vi "test-ramsete.vi"() -> (3 "AtReference End":bool)   [LabVIEW 2019]
uses:
  <vilib>/Rock Robotics/WPI/ThirdParty/JAS_Junk/TrajLib/CHASSIS_SPEEDS.ctl
  <vilib>/Rock Robotics/WPI/ThirdParty/JAS_Junk/TrajLib/POSE2D.ctl
  <vilib>/Rock Robotics/WPI/ThirdParty/JAS_Junk/TrajLib/TRANSLATION2D.ctl
  <vilib>/Rock Robotics/WPI/ThirdParty/JAS_Junk/TrajLib/ROTATION2D.ctl
  <vilib>/Rock Robotics/WPI/ThirdParty/JAS_Junk/TrajLib/TRAJ_STATE.ctl
  <vilib>/Rock Robotics/WPI/ThirdParty/JAS_Junk/TrajLib/TRAJECTORY.ctl
  <vilib>/Rock Robotics/WPI/ThirdParty/JAS_Junk/TrajLib/Rotation_CreateAngle.vi
  <vilib>/Rock Robotics/WPI/ThirdParty/JAS_Junk/TrajLib/Translation_Create.vi
  <vilib>/Rock Robotics/WPI/ThirdParty/JAS_Junk/TrajLib/Trajectory_Library.lvlib
panel:
  out "AtReference":bool
  out "out POSe":T1 {"ROTATION"."SIN" format="%13.4f"; "ROTATION"."COS" format="%13.4f"; "ROTATION"."VALUE" format="%13.4f"; "TRANSLATION"."Y" format="%14.3f"; "TRANSLATION"."X" format="%14.3f"}
  out "TRAJECTORY":T4 {"States"."POSE"."ROTATION"."SIN" format="%13.4f"; "States"."POSE"."ROTATION"."COS" format="%13.4f"; "States"."POSE"."ROTATION"."VALUE" format="%13.4f"; "States"."POSE"."TRANSLATION"."Y" format="%14.3f"; "States"."POSE"."TRANSLATION"."X" format="%14.3f"; "TotalTImeSecs" format="%20.3f"}
  out "OutputTRAJ_STATE":T5={"TimeSeconds"=0.0, "Velocity"=0.0, "Acceleration"=0.0, "POSE"={"TRANSLATION"={"X"=0.0, "Y"=0.0}, "ROTATION"={"VALUE"=0.0, "COS"=1.0, "SIN"=0.0}}, "Curvature"=0.0} {"POSE"."ROTATION"."SIN" format="%13.4f"; "POSE"."ROTATION"."COS" format="%13.4f"; "POSE"."ROTATION"."VALUE" format="%13.4f"; "POSE"."TRANSLATION"."Y" format="%14.3f"; "POSE"."TRANSLATION"."X" format="%14.3f"}
  out "Integer":i32
  out "UpdatedPose":T1 {"ROTATION"."SIN" format="%13.4f"; "ROTATION"."COS" format="%13.4f"; "ROTATION"."VALUE" format="%13.4f"; "TRANSLATION"."Y" format="%14.3f"; "TRANSLATION"."X" format="%14.3f"}
  out "CHASSIS Speeds":T6 {"vOmega" format="%10.3f"; "vY" format="%10.3f"; "vX" format="%10.3f"}
  out "Samp-int":i32
  out "Samp-real":dbl
  # "Ramsete"
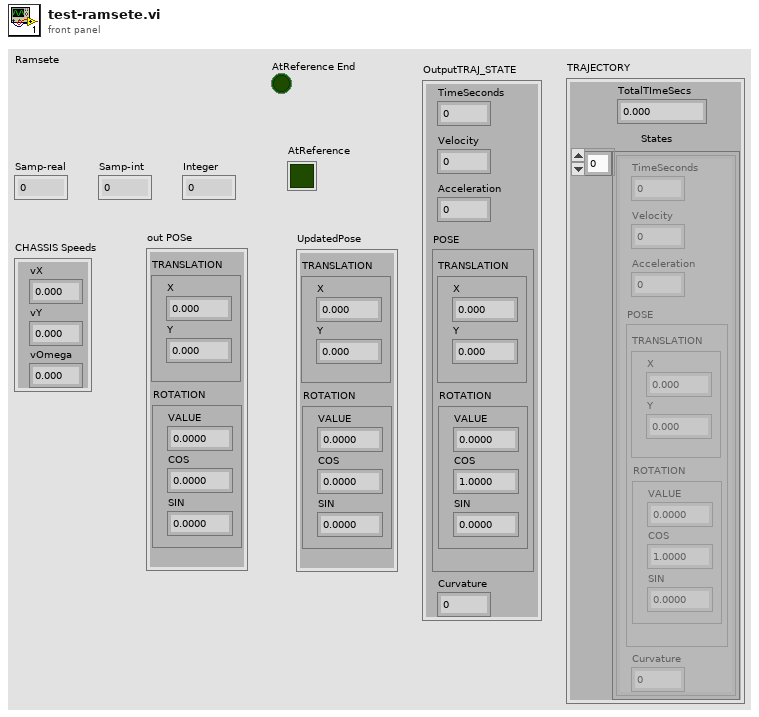
[diagram p1: front panel]
types:
  T1 = typedef "Trajectory_Library.lvlib/POSE2D.ctl" = cluster{"TRANSLATION":T2, "ROTATION":T3}
  T2 = typedef "Trajectory_Library.lvlib/TRANSLATION2D.ctl" = cluster{"X":dbl, "Y":dbl}
  T3 = typedef "Trajectory_Library.lvlib/ROTATION2D.ctl" = cluster{"VALUE":dbl, "COS":dbl, "SIN":dbl}
  T4 = typedef "Trajectory_Library.lvlib/TRAJECTORY.ctl" = cluster{"TotalTImeSecs":dbl, "States":T5[]}
  T5 = typedef "Trajectory_Library.lvlib/TRAJ_STATE.ctl" = cluster{"TimeSeconds":dbl, "Velocity":dbl, "Acceleration":dbl, "POSE":T1, "Curvature":dbl}
  T6 = typedef "Trajectory_Library.lvlib/CHASSIS_SPEEDS.ctl" = cluster{"vX":dbl, "vY":dbl, "vOmega":dbl}
  T7 = typedef "Trajectory_Library.lvlib/TRAJ_CONFIG.ctl" = cluster{"MaxVelocity":dbl, "Max Acceleration":dbl, "StartVelocity":dbl, "End Velocity":dbl, "Reversed":bool, "DiffDrKineConstntDefined":bool, "CentAcellConstntDefined":bool, "DiffDrVoltConstntDefined":bool, "DIFF_DRIVE_KINE_CONSTRAINT":T8, "CENTRIPETAL_ACCEL_CONSTRAINT":T10, "SwerveDrKineConstntDefined":bool, "SWERVE_DRIVE_KINE_CONSTRAINT":T11, "DIFF_DRIVE_VOLTAGE_CONSTRAINT":T14, "MECANUM_DRIVE_KINE_CONSTRAINT":T16, "MecanumDrKineConstntDefined":bool}
  T8 = typedef "Trajectory_Library.lvlib/TRAJ_CONSTRAINT_DIIF_DRIVE_KINEMATICS.ctl" = cluster{"Max Speed (M/S)":dbl, "DIFF_DRIVE_KINEMATICS":T9}
  T9 = typedef "Trajectory_Library.lvlib/DIFF_DRIVE_KINEMATICS.ctl" = cluster{"TrackWidth_Meters":dbl}
  T10 = typedef "Trajectory_Library.lvlib/TRAJ_CONSTRAINT_CENTRIPETAL_ACCEL.ctl" = cluster{"Max Cent Accel":dbl}
  T11 = typedef "Trajectory_Library.lvlib/TRAJ_CONSTRAINT_SWERVE_DRIVE_KINEMATICS.ctl" = cluster{"Max Speed (M/S)":dbl, "SwerveKinematics":T12}
  T12 = typedef "Trajectory_Library.lvlib/SWERVE_DRIVE_KINEMATICS.ctl" = cluster{"NumModules":i32, "InverseKinematics":T13, "ForwardKinematics":T13, "Modules":T2[], "PrevCoR":T2}
  T13 = typedef "NI_Matrix.lvlib/RealMatrix.ctl" = dbl[][]
  T14 = typedef "Trajectory_Library.lvlib/TRAJ_CONSTRAINT_DIIF_DRIVE_VOLTAGE.ctl" = cluster{"Max Voltage":dbl, "DIFF_DRIVE_KINEMATICS":T9, "SIMPLE_MOTOR_FF":T15}
  T15 = typedef "Trajectory_Library.lvlib/SIMPLE_MOTOR_FF.ctl" = cluster{"Ks":dbl, "Kv":dbl, "Ka":dbl}
  T16 = typedef "Trajectory_Library.lvlib/TRAJ_CONSTRAINT_MECA_DRIVE_KINEMATICS.ctl" = cluster{"Max Speed (M/S)":dbl, "MECA_DRIVE_KINEMATICS":T17}
  T17 = typedef "Trajectory_Library.lvlib/MECA_DRIVE_KINEMATICS.ctl" = cluster{"FrontLeft":T2, "FrontRight":T2, "RearLeft":T2, "RearRight":T2, "InverseKinematics":T13, "ForwardKinematics":T13, "PrevCoR":T2}
  T18 = typedef "Trajectory_Library.lvlib/RAMSETE.ctl" = cluster{"B":dbl, "Zeta":dbl, "poseTolerance":T1, "poseError":T1, "Enabled":bool}
  T19 = typedef "Trajectory_Library.lvlib/TWIST2D.ctl" = cluster{"dX":dbl, "dY":dbl, "dTHETA":dbl}
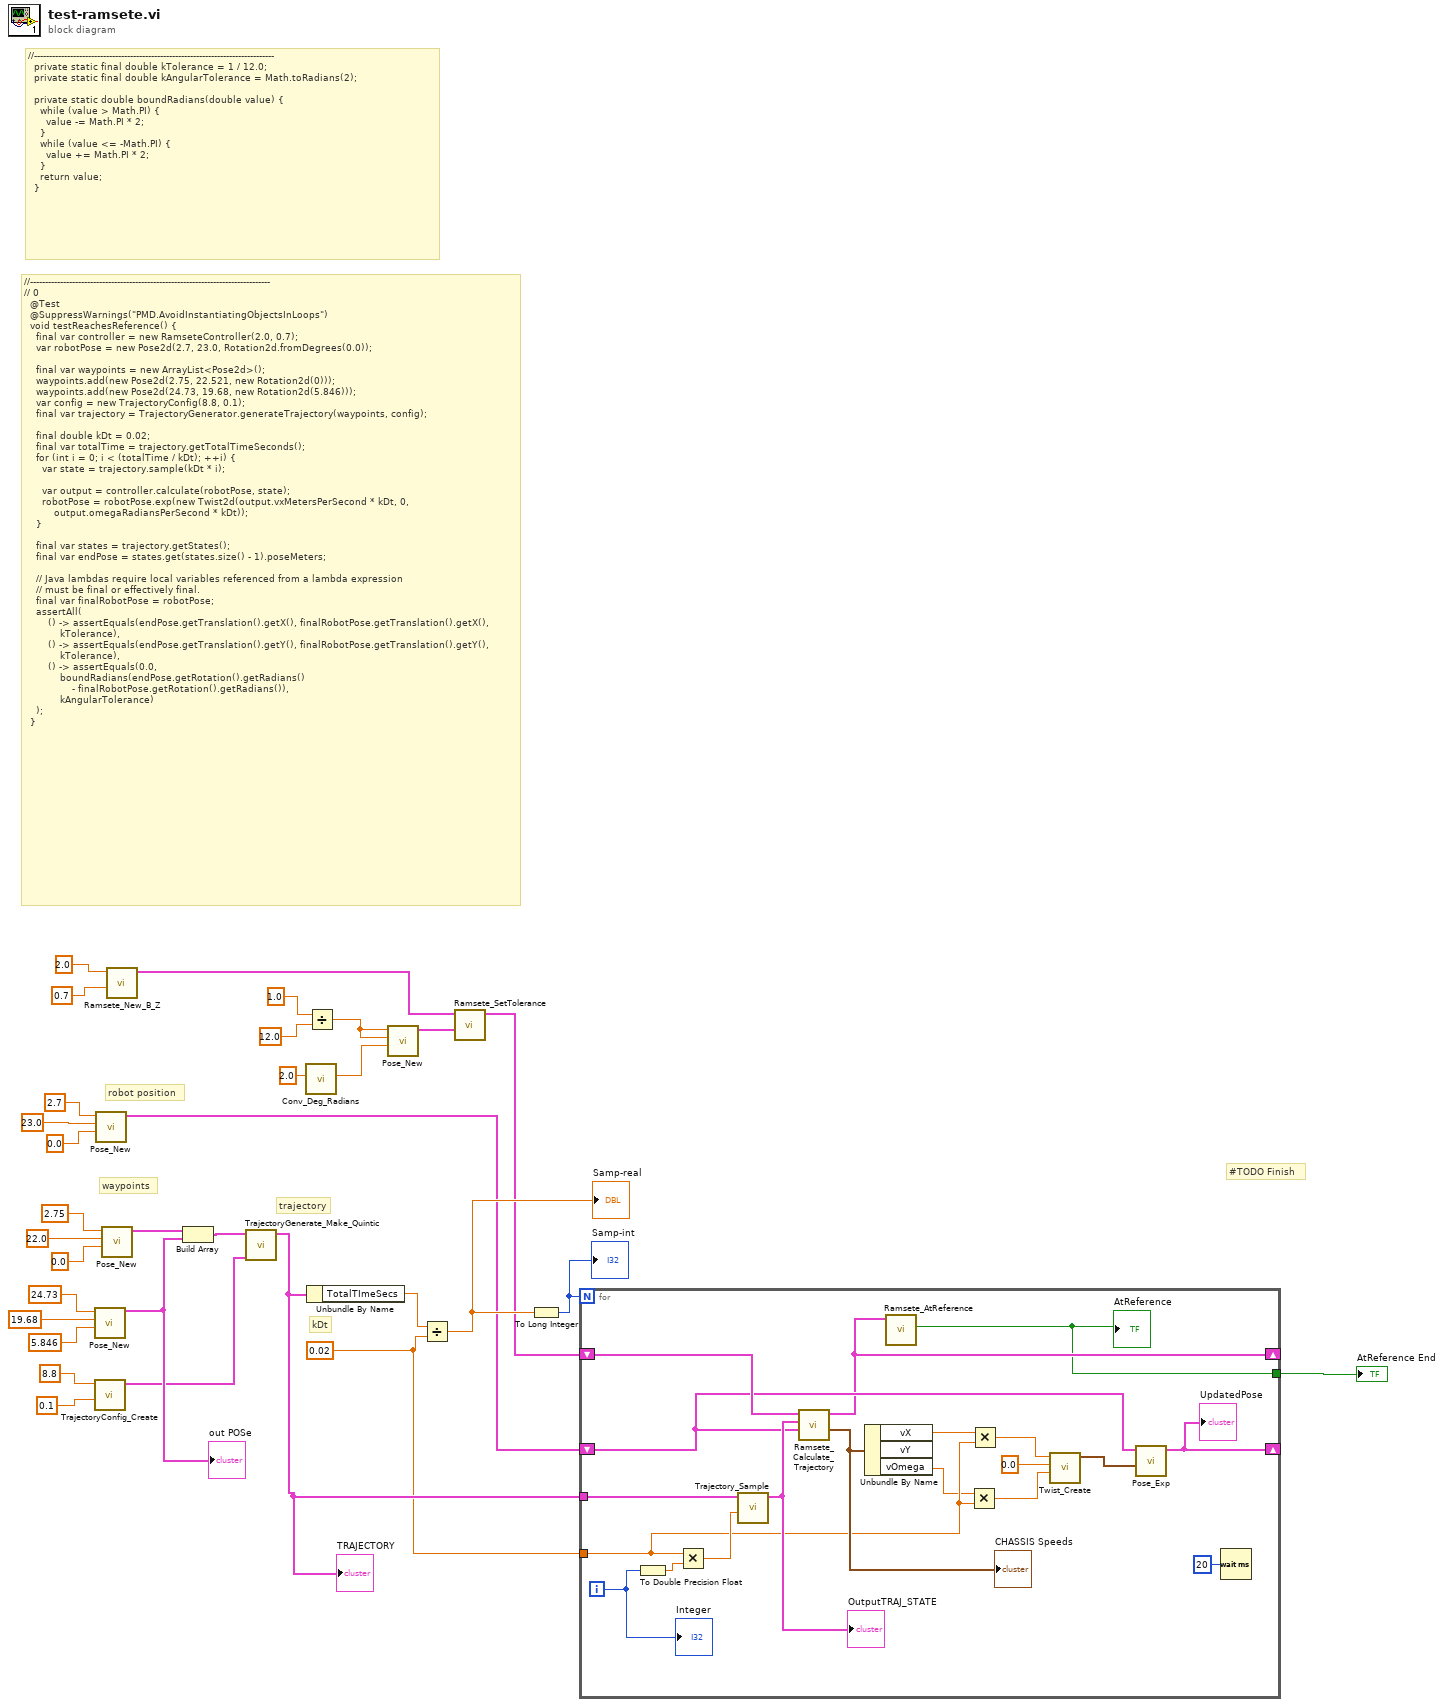
[diagram p0: block diagram]
diagram:
  w10 = 0.02
  # "#TODO Finish"
  # "kDt"
  # "trajectory"
  # "waypoints"
  # "robot position"
  # "//--------------------------------------------------------------------------------\n  private static final double kTolerance = 1 / 12.0;\n  private static final double kAngularTolerance = Math.toRadians(2);\n\n  private static double boundRadians(double value) {\n    while (value > Math.PI) {\n      value -= Math.PI * 2;\n    }\n    while (value <= -Math.PI) {\n      value += Math.PI * 2;\n    }\n    return value;\n  }"
  # "//--------------------------------------------------------------------------------\n// 0\n  @Test\n  @SuppressWarnings(\"PMD.AvoidInstantiatingObjectsInLoops\")\n  void testReachesReference() {\n    final var controller = new RamseteController(2.0, 0.7);\n    var robotPose = new Pose2d(2.7, 23.0, Rotation2d.fromDegrees(0.0));\n\n    final var waypoints = new ArrayList<Pose2d>();\n    waypoints.add(new Pose2d(2.75, 22.521, new Rotation2d(0)));\n    waypoints.add(new Pose2d(24.73, 19.68, new Rotation2d(5.846)));\n    var config = new TrajectoryConfig(8.8, 0.1);\n    final var trajectory = TrajectoryGenerator.generateTrajectory(waypoints, config);\n\n    final double kDt = 0.02;\n    final var totalTime = trajectory.getTotalTimeSeconds();\n    for (int i = 0; i < (totalTime / kDt); ++i) {\n      var state = trajectory.sample(kDt * i);\n\n      var output = controller.calculate(robotPose, state);\n      robotPose = robotPose.exp(new Twist2d(output.vxMetersPerSecond * kDt, 0,\n          output.omegaRadiansPerSecond * kDt));\n    }\n\n    final var states = trajectory.getStates();\n    final var endPose = states.get(states.size() - 1).poseMeters;\n\n    // Java lambdas require local variables referenced from a lambda expression\n    // must be final or effectively final.\n    final var finalRobotPose = robotPose;\n    assertAll(\n        () -> assertEquals(endPose.getTranslation().getX(), finalRobotPose.getTranslation().getX(),\n            kTolerance),\n        () -> assertEquals(endPose.getTranslation().getY(), finalRobotPose.getTranslation().getY(),\n            kTolerance),\n        () -> assertEquals(0.0,\n            boundRadians(endPose.getRotation().getRadians()\n                - finalRobotPose.getRotation().getRadians()),\n            kAngularTolerance)\n    );\n  }"
  n1 = call <vilib>:"Pose_New.vi"("Heading"=5.846, "Y"=19.68, "X"=24.73) -> ("out POSe"=w20:T1)  [unwired: 8 in]
  "out POSe" <- w20
  n2 = call <vilib>:"TrajectoryConfig_Create.vi"("MaxAcceleration"=0.1, "MaxVelocity"=8.8) -> ("TRAJECTORY_CONFIG"=w16:T7)  [unwired: 9 in]
  n3 = call <vilib>:"Pose_New.vi"("Heading"=0.0, "Y"=23.0, "X"=2.7) -> ("out POSe"=w11:T1)  [unwired: 8 in]
  n4 = call <vilib>:"Pose_New.vi"("Heading"=0.0, "Y"=22.0, "X"=2.75) -> ("out POSe"=w21:T1)  [unwired: 8 in]
  n5 = call <vilib>:"Ramsete_New_B_Z.vi"("Zeta"=0.7, "B"=2.0) -> ("outRAMSETE"=w2:T18)  [unwired: 9 in]
  n6 = Build Array(w21, w20) -> (w17:T1[])
  n7 = call <vilib>:"TrajectoryGenerate_Make_Quintic.vi"("traj_config"=w16, "waypointPOSE"=w17) -> ("TRAJECTORY"=w12:T4)  [unwired: 8 in, 1 out]
  "TRAJECTORY" <- w12
  n8 = call <vilib>:"Conv_Deg_Radians.vi"("Degress"=2.0) -> ("Radians"=w5:dbl)  [unwired: 10 in]
  n9 = Divide(x=1.0, y=12.0) -> (x/y=w7:dbl)
  n10 = Unbundle By Name(w12) -> ("TotalTImeSecs"=w15:dbl)
  n11 = call <vilib>:"Pose_New.vi"("Heading"=w5, "Y"=w7, "X"=w7) -> ("out POSe"=w4:T1)  [unwired: 8 in]
  n12 = Divide(x=w15, y=w10) -> (x/y=w13:dbl)
  "Samp-real" <- w13
  n13 = call <vilib>:"Ramsete_SetTolerance.vi"("tolerancePose"=w4, "inRAMSETE"=w2) -> ("outRAMSETE"=w3:T18)  [unwired: 9 in]
  n14 = To Long Integer(number=w13) -> (32bit integer=w14:i32)
  "Samp-int" <- w14
  n15 = for {
    N: w14 -> [_]
    tunnel: w10 -> [w42]
    tunnel: w12 -> [w49]
    shift-right: [w36] -> _
    shift-left: w11 -> [w38]
    shift-right: [w34] -> _
    shift-left: w3 -> [w47]
    tunnel: [w33] -> w1
    i -> [w50]
    n16 = To Double Precision Float(number=w50) -> (double precision float=w51:dbl)
    n17 = Multiply(x=w42, y=w51) -> (x*y=w48:dbl)
    n18 = call <vilib>:"Trajectory_Sample.vi"("Time"=w48, "InputTRAJECTORY"=w49) -> ("OutputTRAJ_STATE"=w46:T5)  [unwired: 9 in]
    "OutputTRAJ_STATE" <- w46
    n19 = call <vilib>:"Ramsete_Calculate_Trajectory.vi"("CurrentPOSE"=w38, "TRAJ_STATE"=w46, "inRAMSETE"=w47) -> ("CHASSIS Speeds"=w45:T6, "outRAMSETE"=w34:T18)  [unwired: 7 in]
    "CHASSIS Speeds" <- w45
    n20 = Unbundle By Name(w45) -> ("vX"=w44:dbl, "vOmega"=w41:dbl)  [unwired: 1 out]
    n21 = call <vilib>:"Ramsete_AtReference.vi"("RAMSETE"=w34) -> ("AtReference"=w33:bool)  [unwired: 10 in]
    "AtReference" <- w33
    n22 = Multiply(x=w41, y=w42) -> (x*y=w39:dbl)
    n23 = Multiply(x=w44, y=w42) -> (x*y=w43:dbl)
    n24 = call <vilib>:"Twist_Create.vi"("dTHETA"=w39, "dY"=0.0, "dX"=w43) -> ("TWIST"=w37:T19)  [unwired: 8 in]
    n25 = call <vilib>:"Pose_Exp.vi"("TWIST"=w37, "POSE"=w38) -> ("UpdatedPose"=w36:T1)  [unwired: 9 in]
    "UpdatedPose" <- w36
    n26 = Wait (ms)(milliseconds to wait=u32 20) -> ()  [unwired: 1 out]
    "Integer" <- w50
  }
  "AtReference End" <- w1
